vi "DN4_CheckEveryChannel'sSamplesCount.vi"(2 "samples count":i32[](array[numeric])) -> (0 "error out":errorcluster)   [LabVIEW 2020]
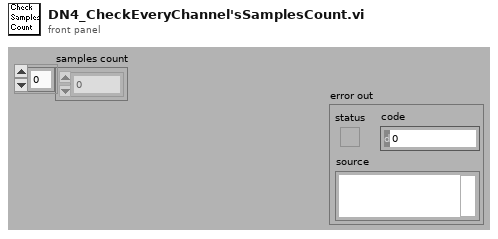
[diagram p1: front panel]
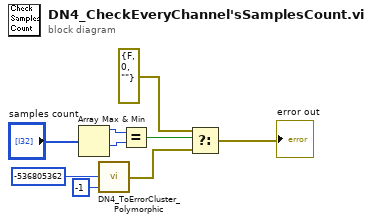
[diagram p0: block diagram]
diagram:
  n1 = Array Max & Min(array="samples count") -> (max value=w6:i32, min value=w2:i32)  [unwired: 2 out]
  n2 = call "DN4_ToErrorCluster_Polymorphic.vi"("task id"=-1, "error code"=-536805362 ("error code (0)")) -> ("error out"=w4:errorcluster)  [unwired: 3 out]
  n3 = Equal?(x=w6, y=w2) -> (x = y?=w7:bool)
  n4 = Select(t=errorcluster {"status"=FALSE, "code"=0, "source"=""}, s=w7, f=w4) -> (s? t:f=→"error out":errorcluster)
